vi "Load Action Core.vi"(8 "error in (no error)":errorcluster, 10 "config file in":T1, 11 "NI DAQmx AI Voltage in":refnum<class "NI DAQmx AI Voltage.lvclass">) -> (0 "error out":errorcluster, 2 "config file out":T1, 3 "NI DAQmx AI Voltage out":refnum<class "NI DAQmx AI Voltage.lvclass">)   [LabVIEW 2023, in "NI DAQmx AI Voltage.lvlib" / "NI DAQmx AI Voltage.lvclass"]
uses:
  NI DAQmx AI Voltage.lvclass
  <vilib>/Utility/config.llb/Config Data RefNum.ctl
  NI DAQmx AI Voltage.lvclass/NI DAQmx AI Voltage.ctl
  <vilib>/Utility/config.llb/NI_LVConfig.lvlib
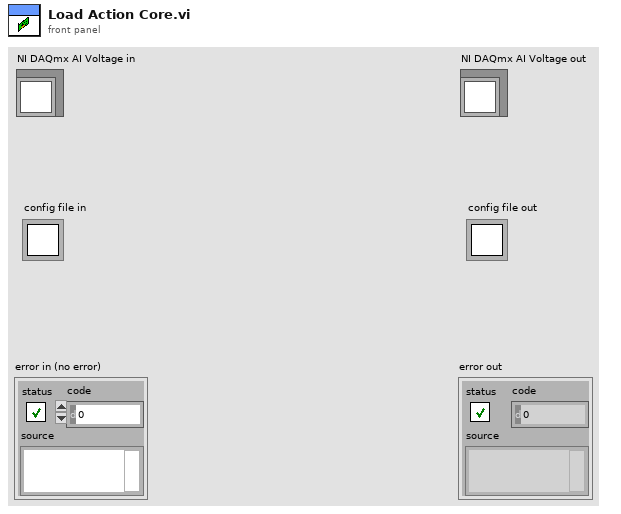
[diagram p1: front panel]
types:
  T1 = typedef "NI_LVConfig.lvlib/Config Data RefNum.ctl" = refnum<k1>
  T2 = cluster{"physical_channels":string, "minimum_value":dbl, "maximum_value":dbl, "sampling_rate":dbl, "samples_per_channel":i32, "clock_source":string}
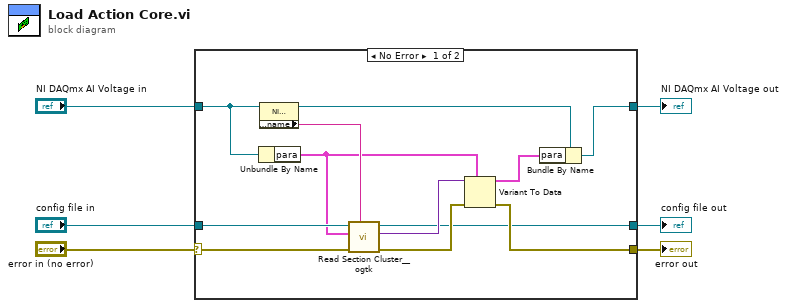
[diagram p0: block diagram]
diagram:
  n1 = case shown="No Error" "error in (no error)" {
    selector: "error in (no error)" -> [w17 w19]
    tunnel: "config file in" -> [w15 w20]
    tunnel: "NI DAQmx AI Voltage in" -> [w18 w21]
    tunnel: [w8 w21] -> w3
    tunnel: [w7 w20] -> w2
    tunnel: [w12 w19] -> w1
    frame No Error {
      n2 = Unbundle By Name(w18) -> ("para"=w9:T2)
      n3 = property class="NI DAQmx AI Voltage.lvclass"(reference=w18) -> (reference out=w11:refnum<class "NI DAQmx AI Voltage.lvclass">, "Accessor:name"=w16:string)  [unwired: 1 in, 1 out]
      n4 = call <userlib>:"Read Section Cluster__ogtk.vi"("section (optional)"=w16, "error in (no error)"=w17, "Section Formatted Cluster Type"=w9, "refnum"=w15) -> ("error out"=w13:errorcluster, "Section Formatted Cluster"=w14:variant, "dup refnum"=w7:T1)  [unwired: 3 in, 2 out]
      n5 = Variant To Data(error in=w13, type=w9, Variant=w14) -> (data=w10:T2, error out=w12:errorcluster)
      n6 = Bundle By Name(cluster=w11, "para"=w10) -> (w8:refnum<class "NI DAQmx AI Voltage.lvclass">)
    }
    frame Error {
    }
  }
  "error out" <- w1
  "NI DAQmx AI Voltage out" <- w3
  "config file out" <- w2
